vi "Write Exports Commit Destination Folder.vi"(8 "error in (no error)":errorcluster, 10 "Exports Commit Destination Folder":path, 11 "Commit in":refnum<class "Commit.lvclass">) -> (0 "error out":errorcluster, 3 "Commit out":refnum<class "Commit.lvclass">)   [LabVIEW 2017, in "CL_G3_VIComponentBuilder.lvlib" / "Commit.lvclass"]
uses:
  Commit.lvclass
  Commit.lvclass/Commit.ctl
  Read Commit Config File.vi
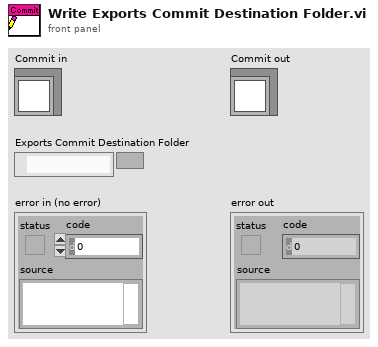
[diagram p1: front panel]
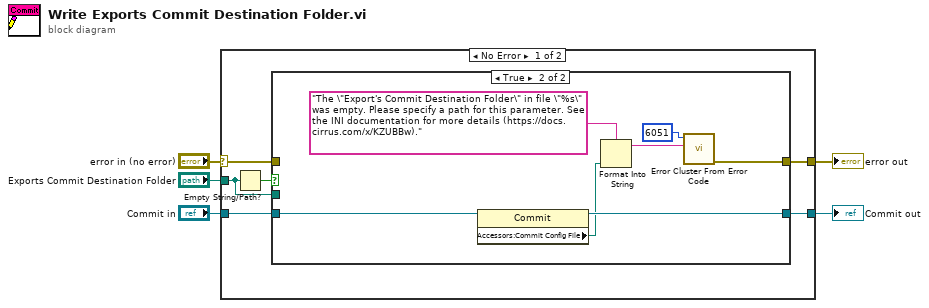
[diagram p0: block diagram]
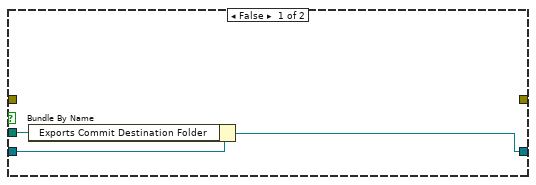
[diagram p2: hidden frame]
diagram:
  n1 = case shown="No Error" "error in (no error)" {
    selector: "error in (no error)" -> [w7 w23]
    tunnel: [w6 w23] -> w4
    tunnel: [w8 w22] -> w3
    tunnel: "Exports Commit Destination Folder" -> [w10 _]
    tunnel: "Commit in" -> [w9 w22]
    frame No Error {
      n2 = Empty String/Path?(string/path=w10) -> (empty?=w11:bool)
      n3 = case shown="True" w11 {
        tunnel: [w14 w20] -> w8
        tunnel: w10 -> [w13 _]
        tunnel: w9 -> [w12 w21]
        tunnel: w7 -> [_ _]
        tunnel: [_ w18] -> w6
        frame False {
          n4 = Bundle By Name(cluster=w12, "Exports Commit Destination Folder"=w13) -> (w14:refnum<class "Commit.lvclass">)
        }
        frame True {
          n5 = property class="Commit"(reference=w21) -> (reference out=w20:refnum<class "Commit.lvclass">, "Accessors:Commit Config File"=w17:path)  [unwired: 1 in, 1 out]
          n6 = Format Into String(format string="The \"Export's Commit Destination Folder\" in file \"%s\" was empty. Please specify a path for this parameter. See the INI documentation for more details (https://docs.cirrus.com/x/KZUBBw).", w17) -> (resulting string=w15:string)  [unwired: 2 in, 1 out]
          n7 = call <vilib>:"Error Cluster From Error Code.vi"("error message (\"\")"=w15, "error code (0)"=6051) -> ("error out"=w18:errorcluster)  [unwired: 7 in]
        }
      }
    }
    frame Error {
    }
  }
  "error out" <- w4
  "Commit out" <- w3
